vi "get_motion_default_speed.vi"(8 "error in (no error)":errorcluster caption="错误输入（无错误）", 11 "OneMotion 输入":refnum<class "OneMotion.lvclass">) -> (0 "error out":errorcluster caption="错误输出", 2 "default speed":i32, 3 "OneMotion 输出":refnum<class "OneMotion.lvclass">)   [LabVIEW 2016, in "MotionControl_UFO_3DOF.lvlib" / "OneMotion.lvclass"]
uses:
  <userlib>/MotionControl_UFO_3DOF/OneMotion/OneMotion.lvclass
  <userlib>/MotionControl_UFO_3DOF/OneMotion/OneMotion.lvclass/OneMotion.ctl
  <userlib>/MotionControl_UFO_3DOF/StepMotor/StepMotor.lvclass/StepMotor.ctl
  <userlib>/MotionControl_UFO_3DOF/StepMotor/StepMotor.lvclass
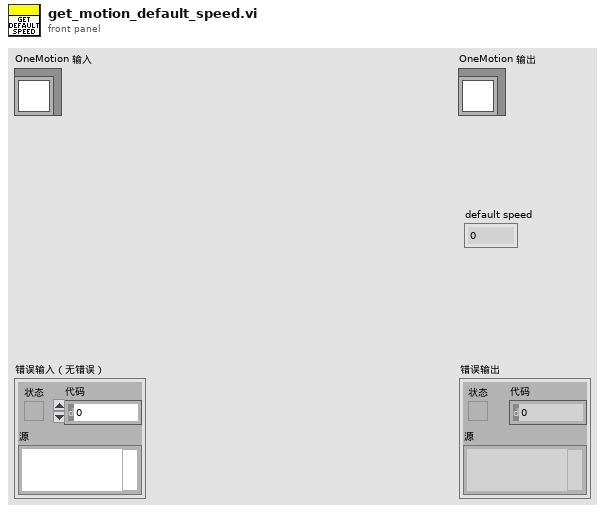
[diagram p1: front panel]
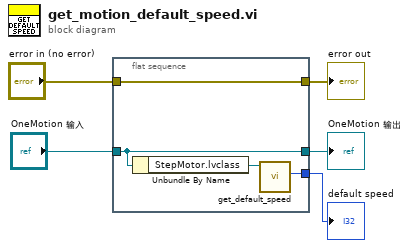
[diagram p0: block diagram]
diagram:
  n1 = flat-sequence {
    tunnel: [w9] -> w5
    tunnel: [w8] -> w3
    tunnel: "OneMotion 输入" -> [w8]
    tunnel: "error in (no error)" -> [w9]
    tunnel: [w6] -> w1
    frame #0 {
      n2 = Unbundle By Name(w8) -> ("StepMotor.lvclass"=w7:refnum<class "StepMotor.lvclass">)
      n3 = call <userlib>:"get_default_speed.vi"("StepMotor输入"=w7) -> ("expected speed"=w6:i32)  [unwired: 8 in, 2 out]
    }
  }
  "error out" <- w5
  "OneMotion 输出" <- w3
  "default speed" <- w1
